vi "Train Magnet (No Objects).vi"(8 "error in (no error)":errorcluster, 11 "Cluster In":T4={"Field"=0.0, "Rate"=0.0, "Status"={"Sweeping"=FALSE, "Clamped"=FALSE, "Hold"=FALSE, "At Rest"=FALSE, "Quench"=FALSE, "Persistent Mode"=FALSE, "Switch Heater"=FALSE}, "ILM Shut Down?"=FALSE, "IO Info"={"Address"={"Com Port"=1, "ISOBUS Address"=2, "GPIB Address"=24, "Communication"=enum."ISOBUS"}, "Version"=enum."IPS"}, "IO Info (Level Meter)"={"Address"={"Com Port"=1, "ISOBUS Address"=5, "GPIB Address"=24, "Communication"=enum."ISOBUS"}, "ILM Name"="", "Display Channel"=[]}, "Training?"=FALSE, "Training Field and Speed Cluster"={"Training Field"=[0.0, 4.108, 5.78, 8.001], "Training Speed"=[0.0057, 0.0022833333333333334, 0.0011333333333333334, 0.0011333333333333334]}}) -> (0 "error out":errorcluster, 2 "This VI":refnum<vi>, 3 "Cluster Out":T4={"Field"=0.0, "Rate"=0.0, "Status"={"Sweeping"=FALSE, "Clamped"=FALSE, "Hold"=FALSE, "At Rest"=FALSE, "Quench"=FALSE, "Persistent Mode"=FALSE, "Switch Heater"=FALSE}, "ILM Shut Down?"=FALSE, "IO Info"={"Address"={"Com Port"=1, "ISOBUS Address"=2, "GPIB Address"=24, "Communication"=enum."ISOBUS"}, "Version"=enum."IPS"}, "IO Info (Level Meter)"={"Address"={"Com Port"=1, "ISOBUS Address"=5, "GPIB Address"=24, "Communication"=enum."ISOBUS"}, "ILM Name"="", "Display Channel"=[]}, "Training?"=FALSE, "Training Field and Speed Cluster"={"Training Field"=[0.0, 4.108, 5.78, 8.001], "Training Speed"=[0.0057, 0.0022833333333333334, 0.0011333333333333334, 0.0011333333333333334]}})   [LabVIEW 2017]
uses:
  Magnet status.ctl
  Oxford/PSSUBS.LLB/PSIO.ctl
  Oxford/BUSGEN.LLB/OxfordAddress.ctl
  Global/Relative Sound Files.vi
  Power Supply.lvclass
panel:
  out "Done":bool
  out "Training":bool
  out "original rate":dbl[unit] caption="Original Rate"
  out "going to field? (false when at field)":bool
  out "going up?":bool
  out "currently going to field":dbl[unit]
  out "current field":dbl[unit]
  out "active":bool
  out "rate":dbl[unit] caption="Current Rate"
  in  "interrupt":bool
  out "Original Field":dbl[unit]
  in  "endprogram":bool
  in  "go":bool
  in  "upanddown":bool=TRUE
  in  "Train to Field":dbl[unit]=7.0
  # "To what field would you like to train the magnet?"
  # "Training means going up to the desired field at the \"train speed\"\nand then coming back down to the starting field, again, at the \"train speed.\" Going to 7 T takes about 42 min, one way."
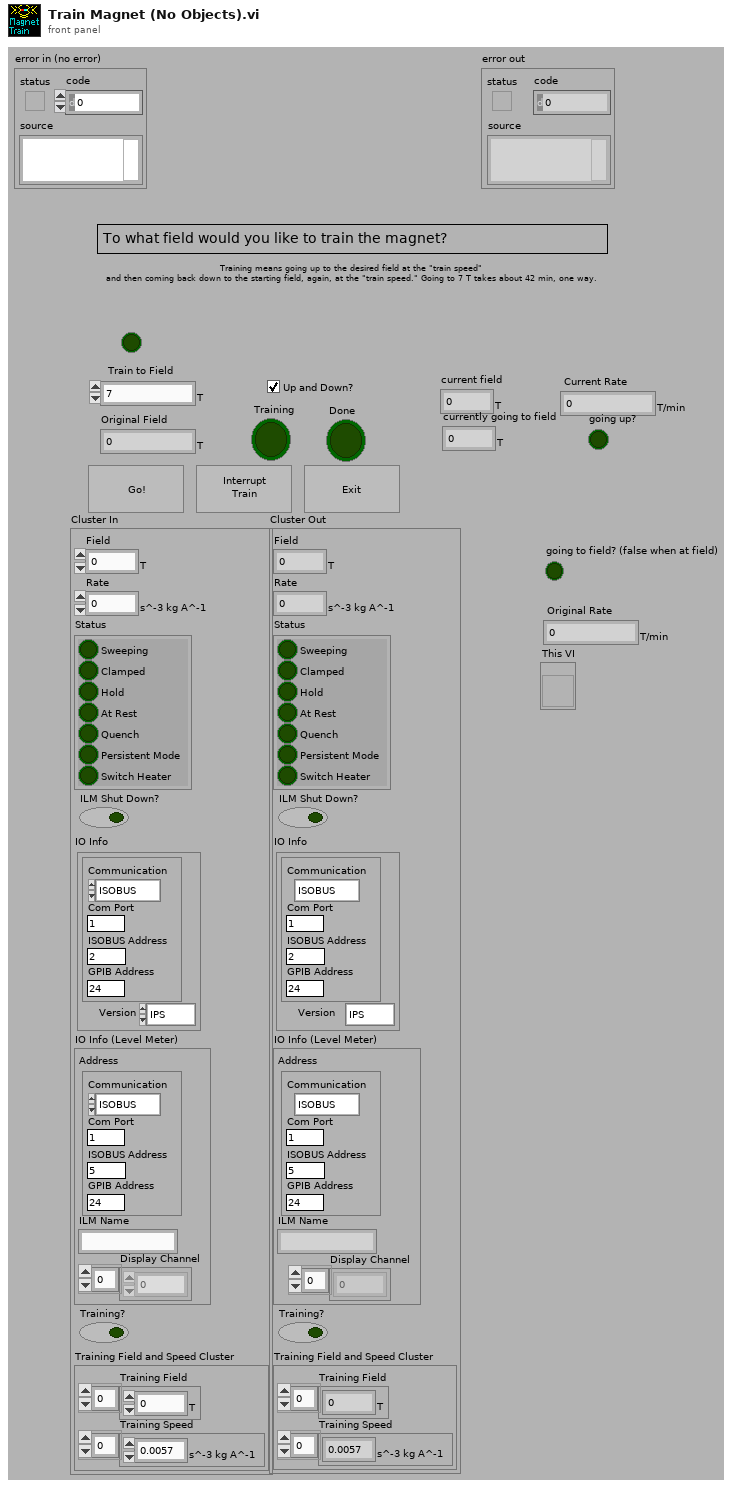
[diagram p1: front panel]
types:
  T1 = typedef "Power Supply.lvclass/Magnet status.ctl" = cluster{"Sweeping":bool, "Clamped":bool, "Hold":bool, "At Rest":bool, "Quench":bool, "Persistent Mode":bool, "Switch Heater":bool}
  T2 = typedef "PSIO.ctl" = cluster{"Address":T3, "Version":enum16{"PS", "IPS"}}
  T3 = typedef "OxfordAddress.ctl" = cluster{"Com Port":i32, "ISOBUS Address":i32, "GPIB Address":i16, "Communication":enum16{"RS232", "ISOBUS", "GPIB", "Gateway"}}
  T4 = cluster{"Field":dbl[unit], "Rate":dbl[unit], "Status":T1, "ILM Shut Down?":bool, "IO Info":T2, "IO Info (Level Meter)":cluster{"Address":T3, "ILM Name":string, "Display Channel":i32[]}, "Training?":bool, "Training Field and Speed Cluster":cluster{"Training Field":dbl[unit][], "Training Speed":dbl[unit][]}}
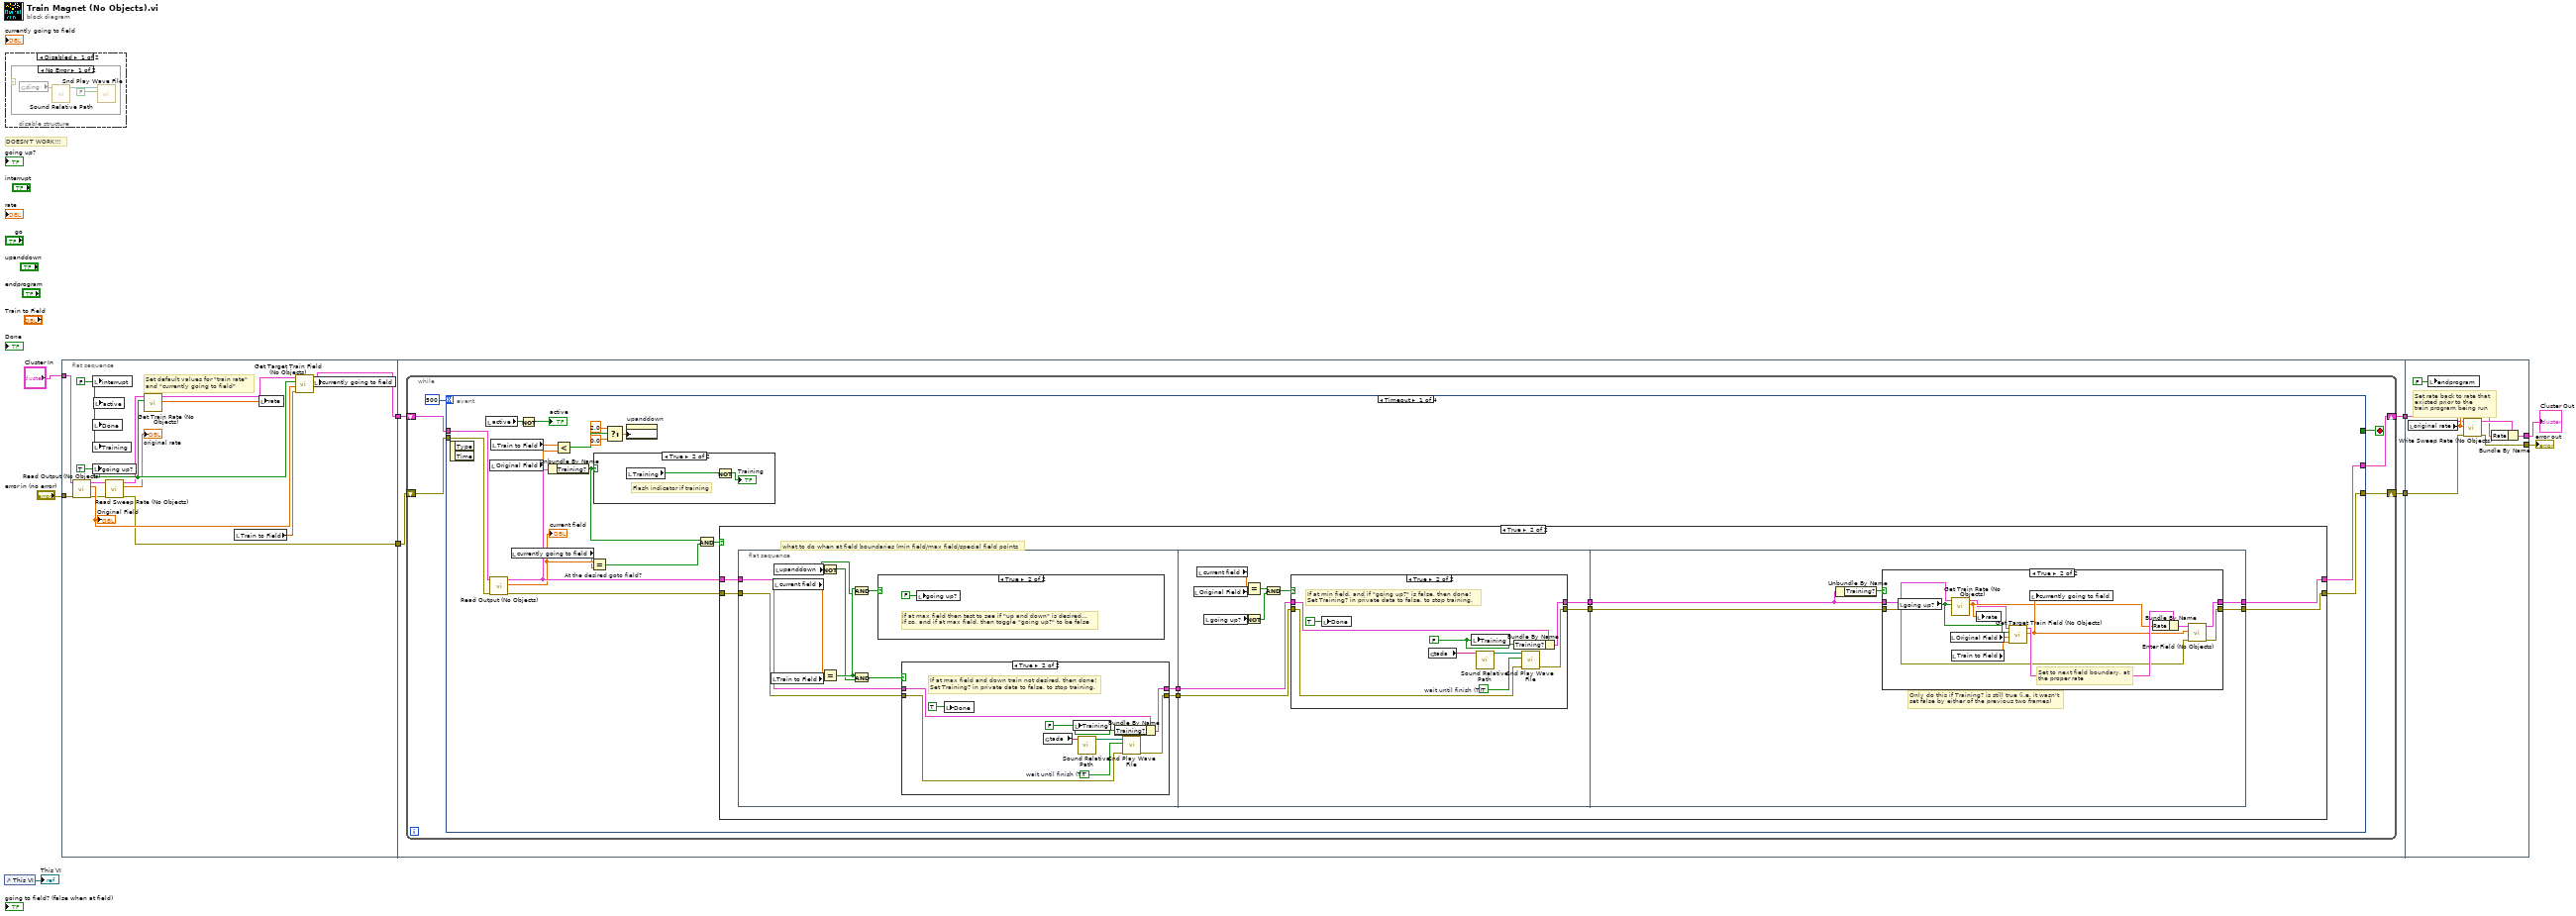
[diagram p0: block diagram]
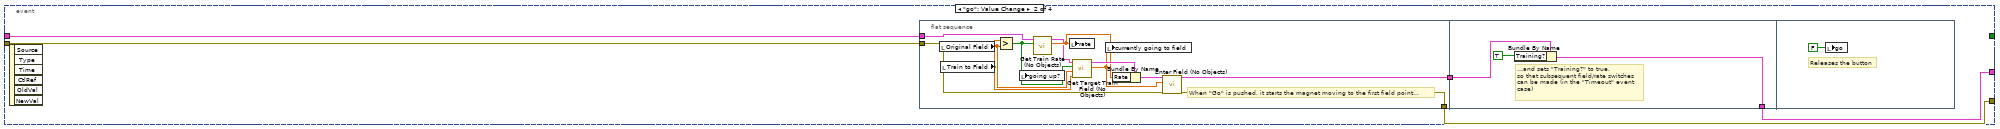
[diagram p10: hidden frame]
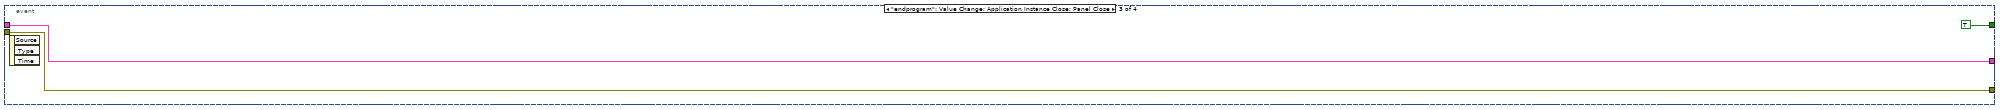
[diagram p11: hidden frame]
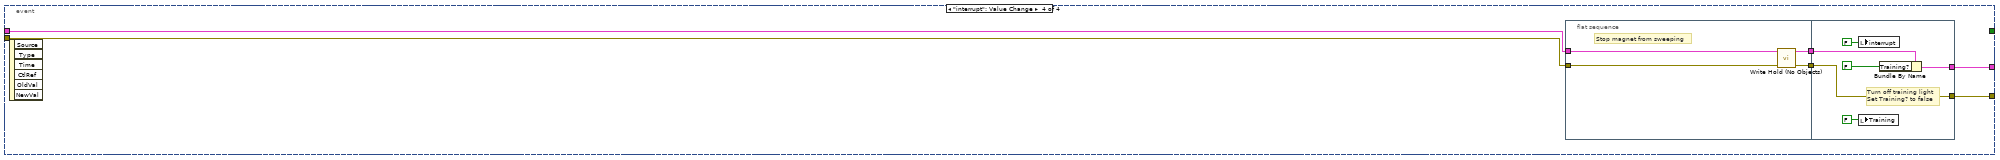
[diagram p12: hidden frame]
diagram:
  # "DOESN'T WORK!!!"
  n1 = control-ref of="This VI"() -> (→"This VI":refnum<vi>)
  n2 = disable-structure shown="Disabled" {
    frame Disabled {
      n3 = case shown="No Error" {
        selector: _ -> [_ _]
        frame No Error {
          n4 = global read "Relative Sound Files.vi" "ding"() -> (w11:string)
          n5 = call "Sound Relative Path.vi"("Sound"=w11) -> ("Relative Path"=w10:path)  [unwired: 10 in]
          n6 = call <vilib>:"Snd Play Wave File.vi"("wait until finish (T)"=FALSE, "wave file path"=w10) -> ()  [unwired: 1 in, 9 out]
        }
        frame Error {
        }
      }
    }
    frame Enabled {
    }
  }
  n7 = flat-sequence {
    tunnel: "Cluster In" -> [w16]
    tunnel: "error in (no error)" -> [w27]
    tunnel: [w22] -> w8
    tunnel: [w20] -> w7
    tunnel: [w31] -> w6
    tunnel: [w30] -> w5
    tunnel: w8 -> [w29]
    tunnel: w7 -> [w28]
    tunnel: w6 -> [w172]
    tunnel: [w177] -> w1
    tunnel: w5 -> [w174]
    tunnel: [w173] -> w4
    frame #0 {
      w25 = TRUE ("going up?")
      w17 = FALSE
      # "Set default values for \"train rate\"\nand \"currently going to field\""
      n8 = call "Read Output (No Objects).vi"("error in (no error)"=w27, "Cluster In"=w16) -> ("error out"=w21:errorcluster, "Field"=w24:dbl[unit], "Cluster Out"=w15:T4)  [unwired: 5 in, 2 out]
      "Original Field" <- w24
      n9 = local write "going up?"(w25) -> ()
      n10 = local write "interrupt"(w17) -> ()
      n11 = local write "Done"(w17) -> ()
      n12 = local write "Training"(w17) -> ()
      n13 = local write "active"(w17) -> ()
      n14 = call "Read Sweep Rate (No Objects).vi"("error in (no error)"=w21, "Cluster In"=w15) -> ("error out"=w20:errorcluster, "Field sweep rate"=→"original rate":dbl[unit], "Cluster Out"=w14:T4)  [unwired: 7 in]
      n15 = call "Get Train Rate (No Objects).vi"("going up?"=w25, "Cluster In"=w14) -> ("Rate Out"=w26:dbl[unit], "Cluster Out"=w13:T4)  [unwired: 8 in]
      n16 = local read "Train to Field"() -> (w23:dbl[unit])
      n17 = local write "rate"(w26) -> ()
      n18 = call "Get Target Train Field (No Objects).vi"("Train to Field"=w23, "Original Field"=w24, "going up?"=w25, "Cluster In"=w13) -> ("Target Field"=w18:dbl[unit], "Cluster Out"=w22:T4)  [unwired: 6 in]
      n19 = local write "currently going to field"(w18) -> ()
    }
    frame #1 {
      n20 = while {
        shift-right: [w34] -> w31
        shift-left: w29 -> [w35]
        shift-right: [w33] -> w30
        shift-left: w28 -> [w32]
        stop <- w37 stop-if-true
        n21 = event shown="[0] Timeout" {
          selector: _ -> [_ _ _ _]
          dyn-events: _ -> [_ _ _ _]
          timeout: 500 -> [_ _ _ _]
          tunnel: [_ _ TRUE ("endprogram") _] -> w37
          tunnel: w35 -> [w38 w135 w155 w161]
          tunnel: [w53 w136 w155 w156] -> w34
          tunnel: [w51 w132 w154 w159] -> w33
          tunnel: w32 -> [w54 w133 w154 w160]
          event Timeout {
            n22 = event-data() -> ()  [unwired: 3 out]
            n23 = local read "active"() -> (w56:bool)
            n24 = local read "Original Field"() -> (w41:dbl[unit])
            n25 = call "Read Output (No Objects).vi"("error in (no error)"=w54, "Cluster In"=w38) -> ("error out"=w52:errorcluster, "Field"=w48:dbl[unit], "Cluster Out"=w50:T4)  [unwired: 5 in, 2 out]
            "current field" <- w48
            n26 = local read "Train to Field"() -> (w42:dbl[unit])
            n27 = local read "currently going to field"() -> (w47:dbl[unit])
            n28 = Not(x=w56) -> (.not. x?=→"active":bool)
            n29 = Unbundle By Name(w50) -> ("Training?"=w45:bool)
            n30 = Less?(x=w42, y=w41) -> (x < y?=w40:bool)
            n31 = Equal? "At the desired goto field?"(x=w48, y=w47) -> (x = y?=w46:bool)
            n32 = case shown="True" w45 {
              frame False {
              }
              frame True {
                # "Flash indicator if training"
                n33 = local read "Training"() -> (w57:bool)
                n34 = Not(x=w57) -> (.not. x?=→"Training":bool)
              }
            }
            n35 = Select(t=2.0 ("f"), s=w40, f=0.0) -> (s? t:f=w39:dbl)
            n36 = property on="upanddown" class="Bool (strict)"("DisabledEnum"=w39) -> ()  [unwired: 2 in, 2 out]
            n37 = And(x=w45, y=w46) -> (x .and. y?=w49:bool)
            n38 = case shown="True" w49 {
              tunnel: w52 -> [w59 w61]
              tunnel: [w59 w68] -> w51
              tunnel: w50 -> [w60 w67]
              tunnel: [w60 w66] -> w53
              frame False {
              }
              frame True {
                # "what to do when at field boundaries (min field/max field/special field points"
                n39 = flat-sequence {
                  tunnel: [w71] -> w65
                  tunnel: w67 -> [w72]
                  tunnel: [w69] -> w62
                  tunnel: w61 -> [w70]
                  tunnel: w65 -> [w95]
                  tunnel: [w94] -> w64
                  tunnel: [w92] -> w63
                  tunnel: w62 -> [w93]
                  tunnel: [w117] -> w66
                  tunnel: [w116] -> w68
                  tunnel: w64 -> [w115]
                  tunnel: w63 -> [w113]
                  frame #0 {
                    n40 = local read "Train to Field"() -> (w78:dbl[unit])
                    n41 = local read "current field"() -> (w79:dbl[unit])
                    n42 = local read "upanddown"() -> (w74:bool)
                    n43 = Not(x=w74) -> (.not. x?=w75:bool)
                    n44 = Equal?(x=w79, y=w78) -> (x = y?=w76:bool)
                    n45 = And(x=w76, y=w74) -> (x .and. y?=w77:bool)
                    n46 = And(x=w76, y=w75) -> (x .and. y?=w73:bool)
                    n47 = case shown="True" w77 {
                      frame False {
                      }
                      frame True {
                        # "if at max field then test to see if \"up and down\" is desired... \nif so, and if at max field, then toggle \"going up?\" to be false"
                        n48 = local write "going up?"(FALSE ("going up?")) -> ()
                      }
                    }
                    n49 = case shown="True" w73 {
                      tunnel: w72 -> [w81 w90]
                      tunnel: [w81 w89] -> w71
                      tunnel: w70 -> [w80 w83]
                      tunnel: [w80 w82] -> w69
                      frame False {
                      }
                      frame True {
                        w86 = TRUE  # wait until finish (T)
                        w87 = FALSE ("Training?")
                        # "If at max field and down train not desired, then done!\nSet Training? in private data to false, to stop training."
                        n50 = local write "Done"(TRUE ("Done")) -> ()
                        n51 = global read "Relative Sound Files.vi" "tada"() -> (w84:string)
                        n52 = local write "Training"(w87) -> ()
                        n53 = call "Sound Relative Path.vi"("Sound"=w84) -> ("Relative Path"=w85:path)  [unwired: 10 in]
                        n54 = Bundle By Name(cluster=w90, "Training?"=w87) -> (w89:T4)
                        n55 = call <vilib>:"Snd Play Wave File.vi"("error in (no error)"=w83, "wait until finish (T)"=w86, "wave file path"=w85) -> ("error out"=w82:errorcluster)  [unwired: 8 out]
                      }
                    }
                  }
                  frame #1 {
                    n56 = local read "Original Field"() -> (w98:dbl[unit])
                    n57 = local read "current field"() -> (w97:dbl[unit])
                    n58 = local read "going up?"() -> (w101:bool)
                    n59 = Equal?(x=w97, y=w98) -> (x = y?=w99:bool)
                    n60 = Not(x=w101) -> (.not. x?=w100:bool)
                    n61 = And(x=w99, y=w100) -> (x .and. y?=w96:bool)
                    n62 = case shown="True" w96 {
                      tunnel: w95 -> [w103 w112]
                      tunnel: [w103 w111] -> w94
                      tunnel: w93 -> [w102 w105]
                      tunnel: [w102 w104] -> w92
                      frame False {
                      }
                      frame True {
                        w108 = TRUE  # wait until finish (T)
                        w109 = FALSE ("Training?")
                        # "If at min field, and if \"going up?\" is false, then done!\nSet Training? in private data to false, to stop training."
                        n63 = local write "Done"(TRUE ("Done")) -> ()
                        n64 = global read "Relative Sound Files.vi" "tada"() -> (w106:string)
                        n65 = local write "Training"(w109) -> ()
                        n66 = call "Sound Relative Path.vi"("Sound"=w106) -> ("Relative Path"=w107:path)  [unwired: 10 in]
                        n67 = Bundle By Name(cluster=w112, "Training?"=w109) -> (w111:T4)
                        n68 = call <vilib>:"Snd Play Wave File.vi"("error in (no error)"=w105, "wait until finish (T)"=w108, "wave file path"=w107) -> ("error out"=w104:errorcluster)  [unwired: 8 out]
                      }
                    }
                  }
                  frame #2 {
                    # "Only do this if Training? is still true (i.e. it wasn't \nset false by either of the previous two frames)"
                    n69 = Unbundle By Name(w115) -> ("Training?"=w114:bool)
                    n70 = case shown="True" w114 {
                      tunnel: w113 -> [w118 w127]
                      tunnel: [w119 w126] -> w117
                      tunnel: [w118 w125] -> w116
                      tunnel: w115 -> [w119 w122]
                      frame False {
                      }
                      frame True {
                        # "Set to next field boundary, at\nthe proper rate"
                        n71 = local read "going up?"() -> (w130:bool)
                        n72 = local read "Original Field"() -> (w128:dbl[unit])
                        n73 = call "Get Train Rate (No Objects).vi"("going up?"=w130, "Cluster In"=w122) -> ("Rate Out"=w123:dbl[unit], "Cluster Out"=w121:T4)  [unwired: 8 in]
                        n74 = local read "Train to Field"() -> (w129:dbl[unit])
                        n75 = local write "rate"(w123) -> ()
                        n76 = call "Get Target Train Field (No Objects).vi"("Train to Field"=w129, "Original Field"=w128, "going up?"=w130, "Cluster In"=w121) -> ("Target Field"=w124:dbl[unit], "Cluster Out"=w131:T4)  [unwired: 6 in]
                        n77 = local write "currently going to field"(w124) -> ()
                        n78 = Bundle By Name(cluster=w131, "Rate"=w123) -> (w120:T4)
                        n79 = call "Enter Field (No Objects).vi"("error in (no error)"=w127, "Target field"=w124, "Cluster In"=w120) -> ("error out"=w125:errorcluster, "Cluster Out"=w126:T4)  [unwired: 7 in]
                      }
                    }
                  }
                }
              }
            }
          }
          event "go": Value Change {
            n80 = event-data() -> ()  [unwired: 7 out]
            n81 = flat-sequence {
              tunnel: [w145] -> w134
              tunnel: [w143] -> w132
              tunnel: w135 -> [w139]
              tunnel: w133 -> [w144]
              tunnel: [w150] -> w136
              tunnel: w134 -> [w149]
              frame #0 {
                # "When \"Go\" is pushed, it starts the magnet moving to the first field point..."
                n82 = local read "Original Field"() -> (w141:dbl[unit])
                n83 = local read "Train to Field"() -> (w142:dbl[unit])
                n84 = Greater?(x=w142, y=w141) -> (0:w140:bool)
                n85 = local write "going up?"(w140) -> ()
                n86 = call "Get Train Rate (No Objects).vi"("going up?"=w140, "Cluster In"=w139) -> ("Rate Out"=w146:dbl[unit], "Cluster Out"=w138:T4)  [unwired: 8 in]
                n87 = local write "rate"(w146) -> ()
                n88 = call "Get Target Train Field (No Objects).vi"("Train to Field"=w142, "Original Field"=w141, "going up?"=w140, "Cluster In"=w138) -> ("Target Field"=w147:dbl[unit], "Cluster Out"=w148:T4)  [unwired: 6 in]
                n89 = local write "currently going to field"(w147) -> ()
                n90 = Bundle By Name(cluster=w148, "Rate"=w146) -> (w137:T4)
                n91 = call "Enter Field (No Objects).vi"("error in (no error)"=w144, "Target field"=w147, "Cluster In"=w137) -> ("error out"=w143:errorcluster, "Cluster Out"=w145:T4)  [unwired: 7 in]
              }
              frame #1 {
                # "...and sets \"Training?\" to true,\nso that subsequent field/rate switches\ncan be made (in the \"Timeout\" event \ncase)"
                n92 = Bundle By Name(cluster=w149, "Training?"=TRUE) -> (w150:T4)
              }
              frame #2 {
                # "Releases the button"
                n93 = local write "go"(FALSE ("go")) -> ()
              }
            }
          }
          event "endprogram": Value Change; Application Instance Close; Panel Close {
            n94 = event-data() -> ()  [unwired: 4 out]
          }
          event "interrupt": Value Change {
            n95 = event-data() -> ()  [unwired: 7 out]
            n96 = flat-sequence {
              tunnel: w161 -> [w162]
              tunnel: w160 -> [w165]
              tunnel: [w164] -> w158
              tunnel: [w163] -> w157
              tunnel: [w171] -> w159
              tunnel: w158 -> [w171]
              tunnel: [w168] -> w156
              tunnel: w157 -> [w167]
              frame #0 {
                # "Stop magnet from sweeping"
                n97 = call "Write Hold (No Objects).vi"("error in (no error)"=w165, "Cluster In"=w162) -> ("error out"=w164:errorcluster, "Cluster Out"=w163:T4)  [unwired: 8 in]
              }
              frame #1 {
                # "Turn off training light\nSet Training? to false"
                n98 = local write "interrupt"(FALSE) -> ()
                n99 = local write "Training"(FALSE ("Training")) -> ()
                n100 = Bundle By Name(cluster=w167, "Training?"=FALSE) -> (w168:T4)
              }
            }
          }
        }
      }
    }
    frame #2 {
      # "Set rate back to rate that\nexisted prior to the \ntrain program being run"
      n101 = local read "original rate"() -> (w175:dbl[unit])
      n102 = local write "endprogram"(FALSE) -> ()
      n103 = call "Write Sweep Rate (No Objects).vi"("error in (no error)"=w174, "rate"=w175, "Cluster In"=w172) -> ("error out"=w173:errorcluster, "Cluster Out"=w176:T4)  [unwired: 7 in]
      n104 = Bundle By Name(cluster=w176, "Rate"=w175) -> (w177:T4)
    }
  }
  "error out" <- w4
  "Cluster Out" <- w1
